vi "Read Address Range.vi"() -> ()   [LabVIEW 2016]
uses:
  Source/GE 5565PIORC/GE 5565PIORC Old.lvclass/GE 5565PIORC Old.ctl
  Source/GE 5565PIORC/VIs/Registers/Local Configuration.Get Register Offset.vi
  Source/GE 5565PIORC/GE 5565PIORC Old.lvclass
panel:
  out "Address Range":u32 format="%.0x"
  in  "VISA resource name":refnum<visa-resource-name>
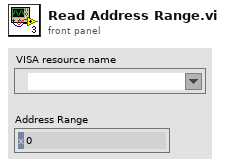
[diagram p1: front panel]
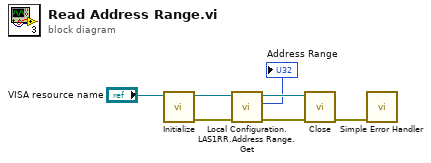
[diagram p0: block diagram]
diagram:
  n1 = call "Initialize.vi"("VISA resource name"="VISA resource name") -> ("error out"=w4:errorcluster, "GE 5565PIORC"=w5:refnum<class "GE 5565PIORC Old.lvclass">)  [unwired: 9 in]
  n2 = call "Local Configuration.LAS1RR.Address Range.Get.vi"("error in (no error)"=w4, "GE 5565PIORC"=w5) -> ("error out"=w2:errorcluster, "Address Range"=→"Address Range":u32, "GE 5565PIORC out"=w3:refnum<class "GE 5565PIORC Old.lvclass">)  [unwired: 7 in]
  n3 = call "Close.vi"("error in (no error)"=w2, "GE 5565PIORC in"=w3) -> ("error out"=w6:errorcluster)  [unwired: 8 in, 1 out]
  n4 = call <vilib>:"Simple Error Handler.vi"("error in (no error)"=w6) -> ()  [unwired: 4 in, 5 out]
